vi "已用时间.vi"() -> ()   [LabVIEW 2014]
panel:
  out "Elapsed Time (s) 2":dbl caption="已用时间(s)"
  out "Elapsed Time (s)":dbl caption="已用时间(s)"
  out "error in (no error) 2":errorcluster caption="error in (no error)"
  in  "error in (no error)":errorcluster caption="错误输入（无错误）"
  in  "停止":bool
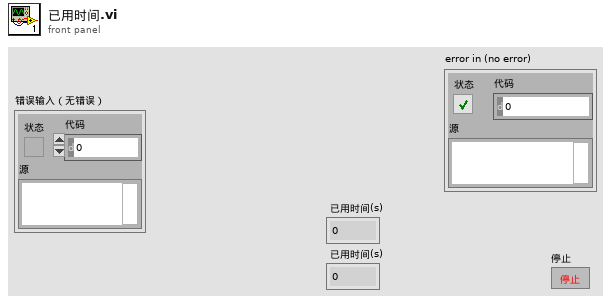
[diagram p1: front panel]
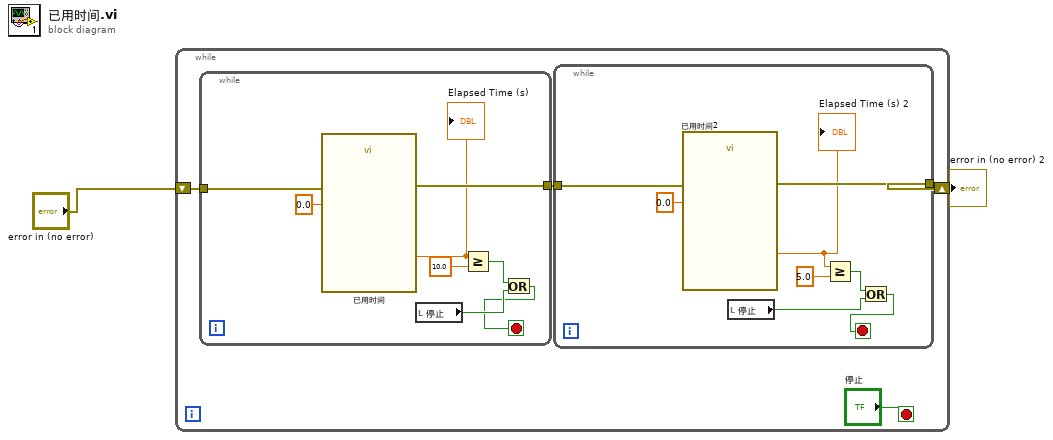
[diagram p0: block diagram]
diagram:
  n1 = while {
    shift-right: [w3] -> w1
    shift-left: "error in (no error)" -> [w5]
    stop <- "停止" stop-if-true
    n2 = while {
      tunnel: w5 -> [w22]
      tunnel: [w21] -> w4
      stop <- w16 stop-if-true
      n3 = call "已用时间"("error in (no error)"=w22, "Set Start Time (s)"=0.0) -> ("Elapsed Time (s)"=w20:dbl, "error out"=w21:errorcluster)  [unwired: 10 in, 6 out]
      "Elapsed Time (s)" <- w20
      n4 = local read "停止"() -> (w17:bool)
      n5 = Greater Or Equal?(x=w20, y=10.0) -> (x >= y?=w18:bool)
      n6 = Or(x=w18, y=w17) -> (x .or. y?=w16:bool)
    }
    n7 = while {
      tunnel: w4 -> [w14]
      tunnel: [w13] -> w3
      stop <- w8 stop-if-true
      n8 = call "已用时间2"("error in (no error)"=w14, "Set Start Time (s)"=0.0) -> ("Elapsed Time (s)"=w12:dbl, "error out"=w13:errorcluster)  [unwired: 10 in, 6 out]
      "Elapsed Time (s) 2" <- w12
      n9 = local read "停止"() -> (w9:bool)
      n10 = Greater Or Equal?(x=w12, y=5.0) -> (x >= y?=w10:bool)
      n11 = Or(x=w10, y=w9) -> (x .or. y?=w8:bool)
    }
  }
  "error in (no error) 2" <- w1
